vi "Single AIN.vi"() -> (0 "error out":errorcluster)   [LabVIEW 2020]
panel:
  out "Value":dbl format="%.6f"
  in  "Name":string="AIN0"
  out "Error String":string
  out "ConnectionType Out":i32
  out "DeviceType Out":i32
  in  "Identifier":string="LJM_idANY"
  in  "ConnectionType":string="LJM_ctANY"
  in  "DeviceType":string="LJM_dtANY"
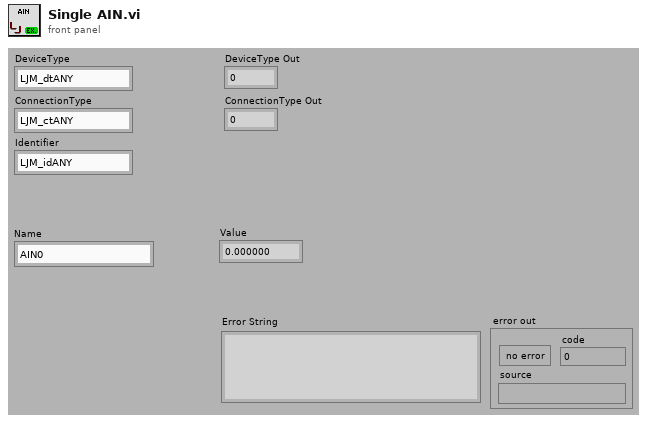
[diagram p1: front panel]
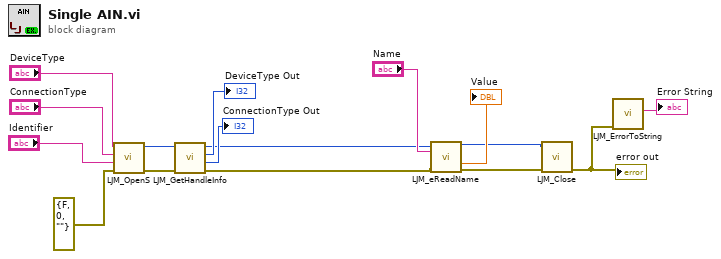
[diagram p0: block diagram]
diagram:
  n1 = call "LJM_OpenS.vi"("error in"=errorcluster {"status"=FALSE, "code"=0, "source"=""} ("error in (no error)"), "Identifier"="Identifier", "ConnectionType"="ConnectionType", "DeviceType"="DeviceType") -> ("error out"=w15:errorcluster, "Handle"=w14:i32)  [unwired: 6 in]
  n2 = call "LJM_GetHandleInfo.vi"("error in"=w15, "Handle In"=w14) -> ("error out"=w3:errorcluster, "ConnectionType"=→"ConnectionType Out":i32, "DeviceType"=→"DeviceType Out":i32, "Handle Out"=w1:i32)  [unwired: 2 in, 4 out]
  n3 = call "LJM_eReadName.vi"("Handle In"=w1, "Name"="Name", "error in"=w3) -> ("Handle Out"=w4:i32, "Value"=→"Value":dbl, "error out"=w2:errorcluster)  [unwired: 10 in]
  n4 = call "LJM_Close.vi"("error in"=w2, "Handle"=w4) -> ("error out"=w8:errorcluster)  [unwired: 9 in]
  "error out" <- w8
  n5 = call "LJM_ErrorToString.vi"("error in"=w8) -> ("String"=→"Error String":string)  [unwired: 10 in]
